vi "Configure Limit.vi"(6 "Fail Action (0:Continue)":i32(ring) items=["Continue", "Stop"], 7 "Enable Limit (Disable)":bool, 8 "error in (no error)":errorcluster, 9 "Upper Limit Value (0)":dbl format="%#_11g", 10 "Lower Limit Value (0)":dbl format="%#_11g", 11 "VISA resource name":refnum<visa-resource-name>) -> (0 "error out":errorcluster, 3 "VISA resource name out":refnum<visa-resource-name>)   [LabVIEW 2020, in "Counter.lvlib" / "PICOTEST U62XXA series.lvlib"]
doc: "Configures the parameters required for post acquisition Limit testing.\n\n<B>Note:</B>\n\nTotalize and Volt Peak Measurements <B>does not</B> support post acquisiton Limit testing.\n\nThe function (OUT*) <B>does not</B> supported on the <B>U6220A</B> model."
uses:
  PICOTEST U62XXA series.lvlib
panel:
  in  "OUT*":u16(ring) items=["OFF", "USB"]
  # "Note: This functionality (OUT*) is  not supported on the U6220 model."
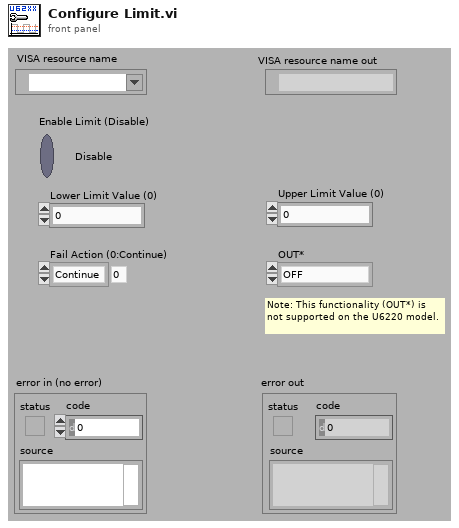
[diagram p1: front panel]
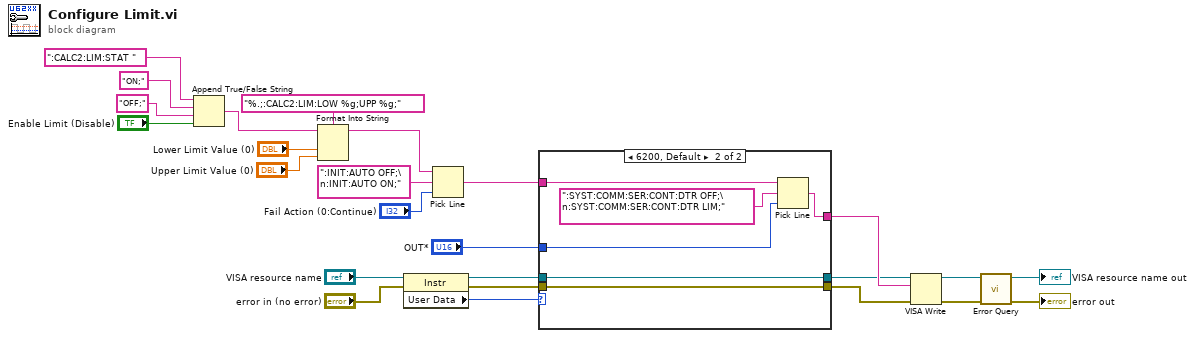
[diagram p0: block diagram]
diagram:
  n1 = Append True/False String(1:"Enable Limit (Disable)", 2:"OFF;" ("false string"), 3:"ON;" ("true string"), 4:":CALC2:LIM:STAT " ("string (\"\")")) -> (0:w18:string)
  n2 = Format Into String(format string="%.;:CALC2:LIM:LOW %g;UPP %g;", initial string=w18, "Lower Limit Value (0)", "Upper Limit Value (0)") -> (resulting string=w13:string)  [unwired: 1 in, 1 out]
  n3 = property class="Instr"(reference="VISA resource name", error in="error in (no error)") -> (reference out=w4:refnum<visa-resource-name>, error out=w3:errorcluster, "User Data"=w10:u32)
  n4 = Pick Line(string ("")=w13, multi-line string=":INIT:AUTO OFF;\n:INIT:AUTO ON;", line index="Fail Action (0:Continue)") -> (output string=w9:string)
  n5 = case shown="6200, Default" w10 {
    tunnel: w9 -> [w28 w33]
    tunnel: [w28 w32] -> w8
    tunnel: "OUT*" -> [_ w31]
    tunnel: w4 -> [w27 w30]
    tunnel: w3 -> [w26 w29]
    tunnel: [w27 w30] -> w2
    tunnel: [w26 w29] -> w1
    frame 6220 {
      # "U6220A does not support OUT* USB"
    }
    frame 6200, Default {
      n6 = Pick Line(string ("")=w33, multi-line string=":SYST:COMM:SER:CONT:DTR OFF;\n:SYST:COMM:SER:CONT:DTR LIM;", line index=w31) -> (output string=w32:string)
    }
  }
  n7 = VISA Write(VISA resource name=w2, write buffer=w8, error in (no error)=w1) -> (VISA resource name out=w7:refnum<visa-resource-name>, error out=w6:errorcluster)  [unwired: 1 out]
  n8 = call "Error Query.vi"("error in (no error)"=w6, "VISA resource name"=w7) -> ("error out"=→"error out":errorcluster, "VISA resource name out"=→"VISA resource name out":refnum<visa-resource-name>)  [unwired: 6 in, 2 out]
